vi "Whole Brain Imaging v14.vi"() -> ()   [LabVIEW 2013]
doc: "v4: Added NI DAQ board instead of LabJack\n\nv5: Modified autofocus routine. Changed to triangle wave - AUTOFOCUS DOES NOT WORK ANYMORE\n\nv6: Modified autofocus to work with Triangle Wave. Added Saved Image Number to Lab Jack String."
uses:
  <vilib>/Platform/TimedLoop/XDataNode/timing_clust.ctl
  <vilib>/Platform/TimedLoop/XDataNode/nitl_modes.ctl
  <vilib>/Platform/TimedLoop/XDataNode/wakeup.ctl
  <vilib>/addons/Multicore Analysis and Sparse Matrix/Signal Operation/_sigop/Algorithm Domain.ctl
  <vilib>/event_ctls.llb/eventvkey.ctl
  <vilib>/DAQmx/read.llb/DAQmx Read (Analog 1D DBL NChan 1Samp).vi
  <vilib>/DAQmx/write.llb/DAQmx Write (Analog DBL 1Chan 1Samp).vi
  <vilib>/DAQmx/miscellaneous.llb/DAQmx Fill In Error Info.vi
  <vilib>/addons/Multicore Analysis and Sparse Matrix/Signal Operation/_sigop/1D Convolution (DBL).vi
  <vilib>/addons/Multicore Analysis and Sparse Matrix/Statistics/_statistics/Mean (DBL).vi
  <vilib>/platform/TimedLoop/XDataNode/XDataNode.xnode
  <vilib>/Platform/TimedLoop/XDataNode/XDNodeRunTimeDep.lvlib
  <vilib>/Analysis/NI_AALBase.lvlib
  <vilib>/addons/Multicore Analysis and Sparse Matrix/Signal Operation/NI_MASM_SigOperation.lvlib
  <vilib>/addons/Multicore Analysis and Sparse Matrix/Statistics/NI_MASM_Statistics.lvlib
panel:
  out "Full Cycle 2":dbl[](graph)=[4.263103829970631, 4.263103829970631, 4.263103829970631, 4.263103829970631, 4.263103829970631, 4.263103829970631, 4.263103829970631, 4.263103829970631, 4.263103829970631, 4.263103829970631, 4.263103829970631, 4.263103829970631, 4.263103829970631, 4.263103829970631, 4.263103829970631, 4.263103829970631, 4.263103829970631, 4.263103829970631, 4.263103829970631, 4.263103829970631, 4.263103829970631, 4.263103829970631, 4.263103829970631, 4.263103829970631, 4.263103829970631, 4.263103829970631, 4.263103829970631, 4.263103829970631, 4.263103829970631, 4.263103829970631, 4.263103829970631, 4.263103829970631, 4.263103829970631, 4.263103829970631, 4.263103829970631, 4.263103829970631, 4.263103829970631, 4.263103829970631, 4.263103829970631, 4.263103829970631, 4.263103829970631, 4.263103829970631, 4.263103829970631, 4.263103829970631, 4.263103829970631, 4.263103829970631, 4.263103829970631, 4.263103829970631, 4.263103829970631, 4.263103829970631, 4.263103829970631, 4.263103829970631, 4.263103829970631, 4.263103829970631, 4.263103829970631, 4.263103829970631, 4.263103829970631, 4.263103829970631, 4.263103829970631, 4.263103829970631, 4.263103829970631, 4.263103829970631, 4.263103829970631, 4.263103829970631, 4.263103829970631, 4.263103829970631, 4.263103829970631, 4.263103829970631]
  out "output cluster 2":T1
  out "loopdiff2":i64
  out "output cluster":T2
  in  "Frames 2 wait":i32=1000
  out "Slide":i32(slide) max=1000 scale=-1.0..1000.0
  in  "Latency Check":bool
  out "photodiode":dbl
  in  "Set amplitude":bool
  out "Current Z-ramp Amplitude":dbl=4.0 format="%_3g"
  in  "Focus Knob COM Port":refnum<visa-resource-name>="COM7"
  out "Motorized Focus Knob Found":bool
  out "Turn Up (Counterclockwise)":bool
  out "Turn Down (Clockwise)":bool
  in  "Target Trim (Frames)":dbl
  out "Full Cycle":dbl[](graph)=[4.263103829970631, 4.263103829970631, 4.263103829970631, 4.263103829970631, 4.263103829970631, 4.263103829970631, 4.263103829970631, 4.263103829970631, 4.263103829970631, 4.263103829970631, 4.263103829970631, 4.263103829970631, 4.263103829970631, 4.263103829970631, 4.263103829970631, 4.263103829970631, 4.263103829970631, 4.263103829970631, 4.263103829970631, 4.263103829970631, 4.263103829970631, 4.263103829970631, 4.263103829970631, 4.263103829970631, 4.263103829970631, 4.263103829970631, 4.263103829970631, 4.263103829970631, 4.263103829970631, 4.263103829970631, 4.263103829970631, 4.263103829970631, 4.263103829970631, 4.263103829970631, 4.263103829970631, 4.263103829970631, 4.263103829970631, 4.263103829970631, 4.263103829970631, 4.263103829970631, 4.263103829970631, 4.263103829970631, 4.263103829970631, 4.263103829970631, 4.263103829970631, 4.263103829970631, 4.263103829970631, 4.263103829970631, 4.263103829970631, 4.263103829970631, 4.263103829970631, 4.263103829970631, 4.263103829970631, 4.263103829970631, 4.263103829970631, 4.263103829970631, 4.263103829970631, 4.263103829970631, 4.263103829970631, 4.263103829970631, 4.263103829970631, 4.263103829970631, 4.263103829970631, 4.263103829970631, 4.263103829970631, 4.263103829970631, 4.263103829970631, 4.263103829970631]
  out "Peak Position":dbl=nan
  out "Target":dbl=17.0
  in  "AutoFocus":u16(ring)=1 items=["Both", "Red", "Green"]
  out "Stage Y":i32=-50106
  out "Stage X":i32=-79365
  out "TotalFramesHidden":i32=32650
  out "Half Cycle":dbl[](graph)
  out "Saved Images Hidden":i32=28989
  in  "Z Ramp\nFrequency (Hz)\n[Must Quit To Update]":dbl=3.0
  in  "Latency Shift (Frames)":i16 max=5000 step=1
  out "sCMOS Image":u16[][](graph)
  in  "ROI":T3={"Horizontal Offset"=418, "Vertical Offset"=818, "Horizontal Width"=1200, "Vertical Width"=600}
  in  "Exposure (ms)":dbl=5.0
  in  "Binning":u16(ring)=1 items=["1x1"=1, "2x2"=2, "4x4"=4]
  out "Read Frames":i32=32581
  in  "Save Image":bool
  out "Written":string="\r\r---------------------  NEW FILE  ---------------------\rO:\\20150616\\BrainScanner20150616_111602\r\r6/16/2015 11:17 AM\rignore first 17000 frames\n\r\r6/16/2015 11:17 AM\runtil third flash\n\r\r6/16/2015 11:18 AM\rbecause my autofocus gain was off\n\r\r6/16/2015 11:18 AM\rworm isn't very active\n\r\r"
  in  "Comments":string
  out "User Comments  File":path=path "O:/20150616/Comments.txt"
  in  "Zero DC Offset":bool
  out "Quit Pushed?":bool=TRUE
  in  "Autofocus Gain":dbl=0.03
  out "Camera Trigger":dbl=0.00885779825410911 format="%.6f"
  out "Camera Frame File":path=path "O:/20150616/BrainScanner20150616_111602/CameraFrameData.txt"
  out "FxnGen Sync":dbl=0.14061238584404193 format="%.6f"
  out "Z Sensor":dbl=6.145352387169191 format="%.6f"
  out "LabJack File":path=path "O:/20150616/BrainScanner20150616_111602/LabJackData.txt"
  out "Dropped Frames":i32=68
  out "Current Image":u16[][](array[numeric])
  out "Image StDev":dbl=4.263103829970631
  out "FuncGen Voltage":dbl=5.836089361558744 format="%.6f"
  out "Z-ramp DC Offset":dbl=nan
  in  "Autofocus":bool
  out "sCMOS Camera Image File":path=path "O:/20150616/BrainScanner20150616_111602/sCMOS_Frames_U16_1024x1024.dat"
  in  "Z-ramp":bool
  in  "Z-ramp Amplitude (4) (Votls)":dbl=4.0 format="%_3g"
  out "Elapsed Time":string="0 : 2 : 43.5"
  out "Saved Frames":i32=28988
  out "Save Directory":path=path "O:/20150616/BrainScanner20150616_111602"
  out "Camera Info":string="C11440-22C; S/N: 751007; 2.50.A"
  out "Total Frames":i32=32649
  in  "Quit":bool
  # "Note: For unknwon reasons, the latency varies from session-to-session and also varies with sweep frequency.\nTo measure and compensate for the latency:\n1) Set Gain to 0 and turn on autofocus.\n2) While recording from bead slide,  adjust  focus knob so that only one peak appears in Full Cycle graph. Beads should be at extreme edge of scan range.\n3)Adjust the latency shift until the single peak appears split on both sides of the graph. \n4) Adjust the focus knob so the beads are back in the center of the scan range\n5) Make the autofocus gain non-zero (e.g. 0.1). You will likely need to try both positive and negative values."
  # "ChangeLog:\nv14. Andy tries to add in the  focus knob controller"
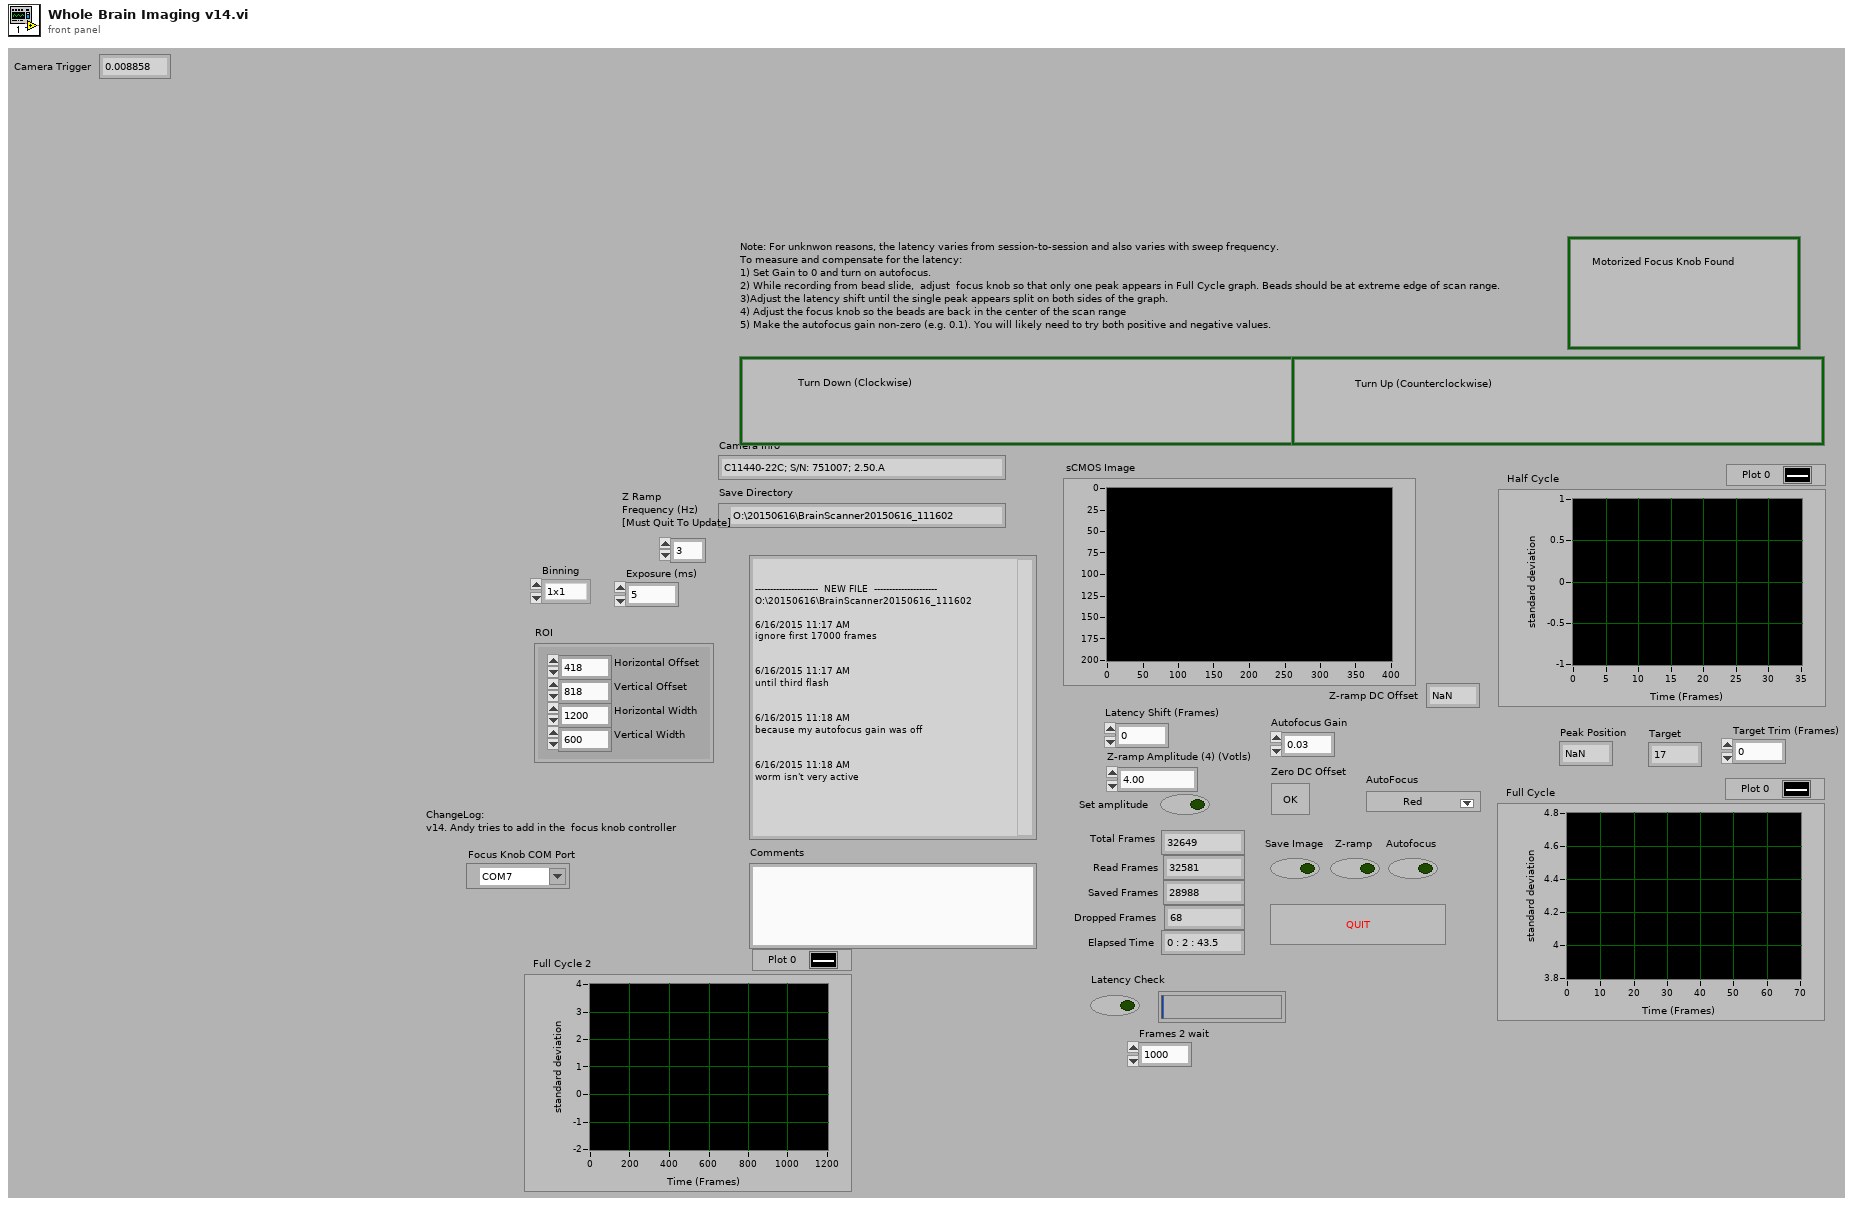
[diagram p1: front panel]
types:
  T1 = cluster{"Waveform":dbl, "standard deviation":dbl}
  T2 = cluster{"Actual Start [i]":i64, "standard deviation":dbl}
  T3 = cluster{"Horizontal Offset":i32, "Vertical Offset":i32, "Horizontal Width":i32, "Vertical Width":i32}
  T4 = enum8{"Enabled", "Disabled", "Disabled and Grayed Out"}
  T5 = typedef "XDNodeRunTimeDep.lvlib/timing_clust.ctl" = cluster{"Expected End [f-1]":u64, "Actual End [f-1]":u64, "Finished Late? [f-1]":bool, "Expected End [i-1]":u64, "Actual End [i-1]":u64, "Finished Late? [i-1]":bool, "Expected Start [i]":u64, "Actual Start [i]":u64, "Expected Start [f]":u64, "Actual Start [f]":u64, "Source Name":string, "Structure Name":string, "Period":i64, "Deadline":i64, "Offset":i64, "Start":i64, "Priority":i32, "Timeout":i32, "Mode":T6, "Wakeup Reason":T7, "Error":errorcluster, "Source Type":string, "Secondary Source Type":string, "Global End Time":u64, "Global Start Time":u64, "Frame Duration":u64, "Iteration Duration":u64, "Assigned CPU":i32, "I/O Scan Engine Mode":u32}
  T6 = typedef "XDNodeRunTimeDep.lvlib/nitl_modes.ctl" = enum32{"No Change", "Process missed periods, maintain original phase", "Discard missed periods, maintain original phase", "Process missed periods, ignore original phase", "Discard missed periods, ignore original phase"}
  T7 = typedef "XDNodeRunTimeDep.lvlib/wakeup.ctl" = enum32{"Normal", "Aborted", "Asynchronous wakeup", "Timing source error", "Timed loop error", "Timeout"}
  T8 = typedef "NI_MASM_SigOperation.lvlib/Algorithm Domain.ctl" = i32
  T9 = enum16{"open", "replace", "create", "open or create", "replace or create", "replace or create with confirmation"}
  T10 = cluster{"height":u32, "width":u32, "datatype":u32}
  T11 = cluster{"Mode":u32, "Polarity":u32, "Period":dbl, "Delay":dbl}
  T12 = typedef "eventvkey.ctl" = enum16{"ASCII", "Enter", "Return", "Shift", "Ctrl", "Alt", "Cmd", "Opt", "Caps", "NumLock", "Clear", "Break", "Up", "Down", "Left", "Right", "Insert", "Delete", "Home", "End", "PageUp", "PageDown", "Escape", "Help", "Pause", "ScrollLock", "F1", "F2", "F3", "F4", "F5", "F6", "F7", "F8", "F9", "F10", "F11", "F12", "F13", "F14", "F15", "F16", "F17", "F18", "F19", "F20", "F21", "F22", "F23", "F24", "Play", "VolumeUp", "VolumeDown", "Mute", "Two Byte Char"}
  T13 = enum16{"big-endian, network order", "native, host order", "little-endian"}
  T14 = cluster{"standard deviation":dbl, "Waveform":dbl}
  T15 = cluster{"millisecond timer value":u32, "standard deviation":dbl}
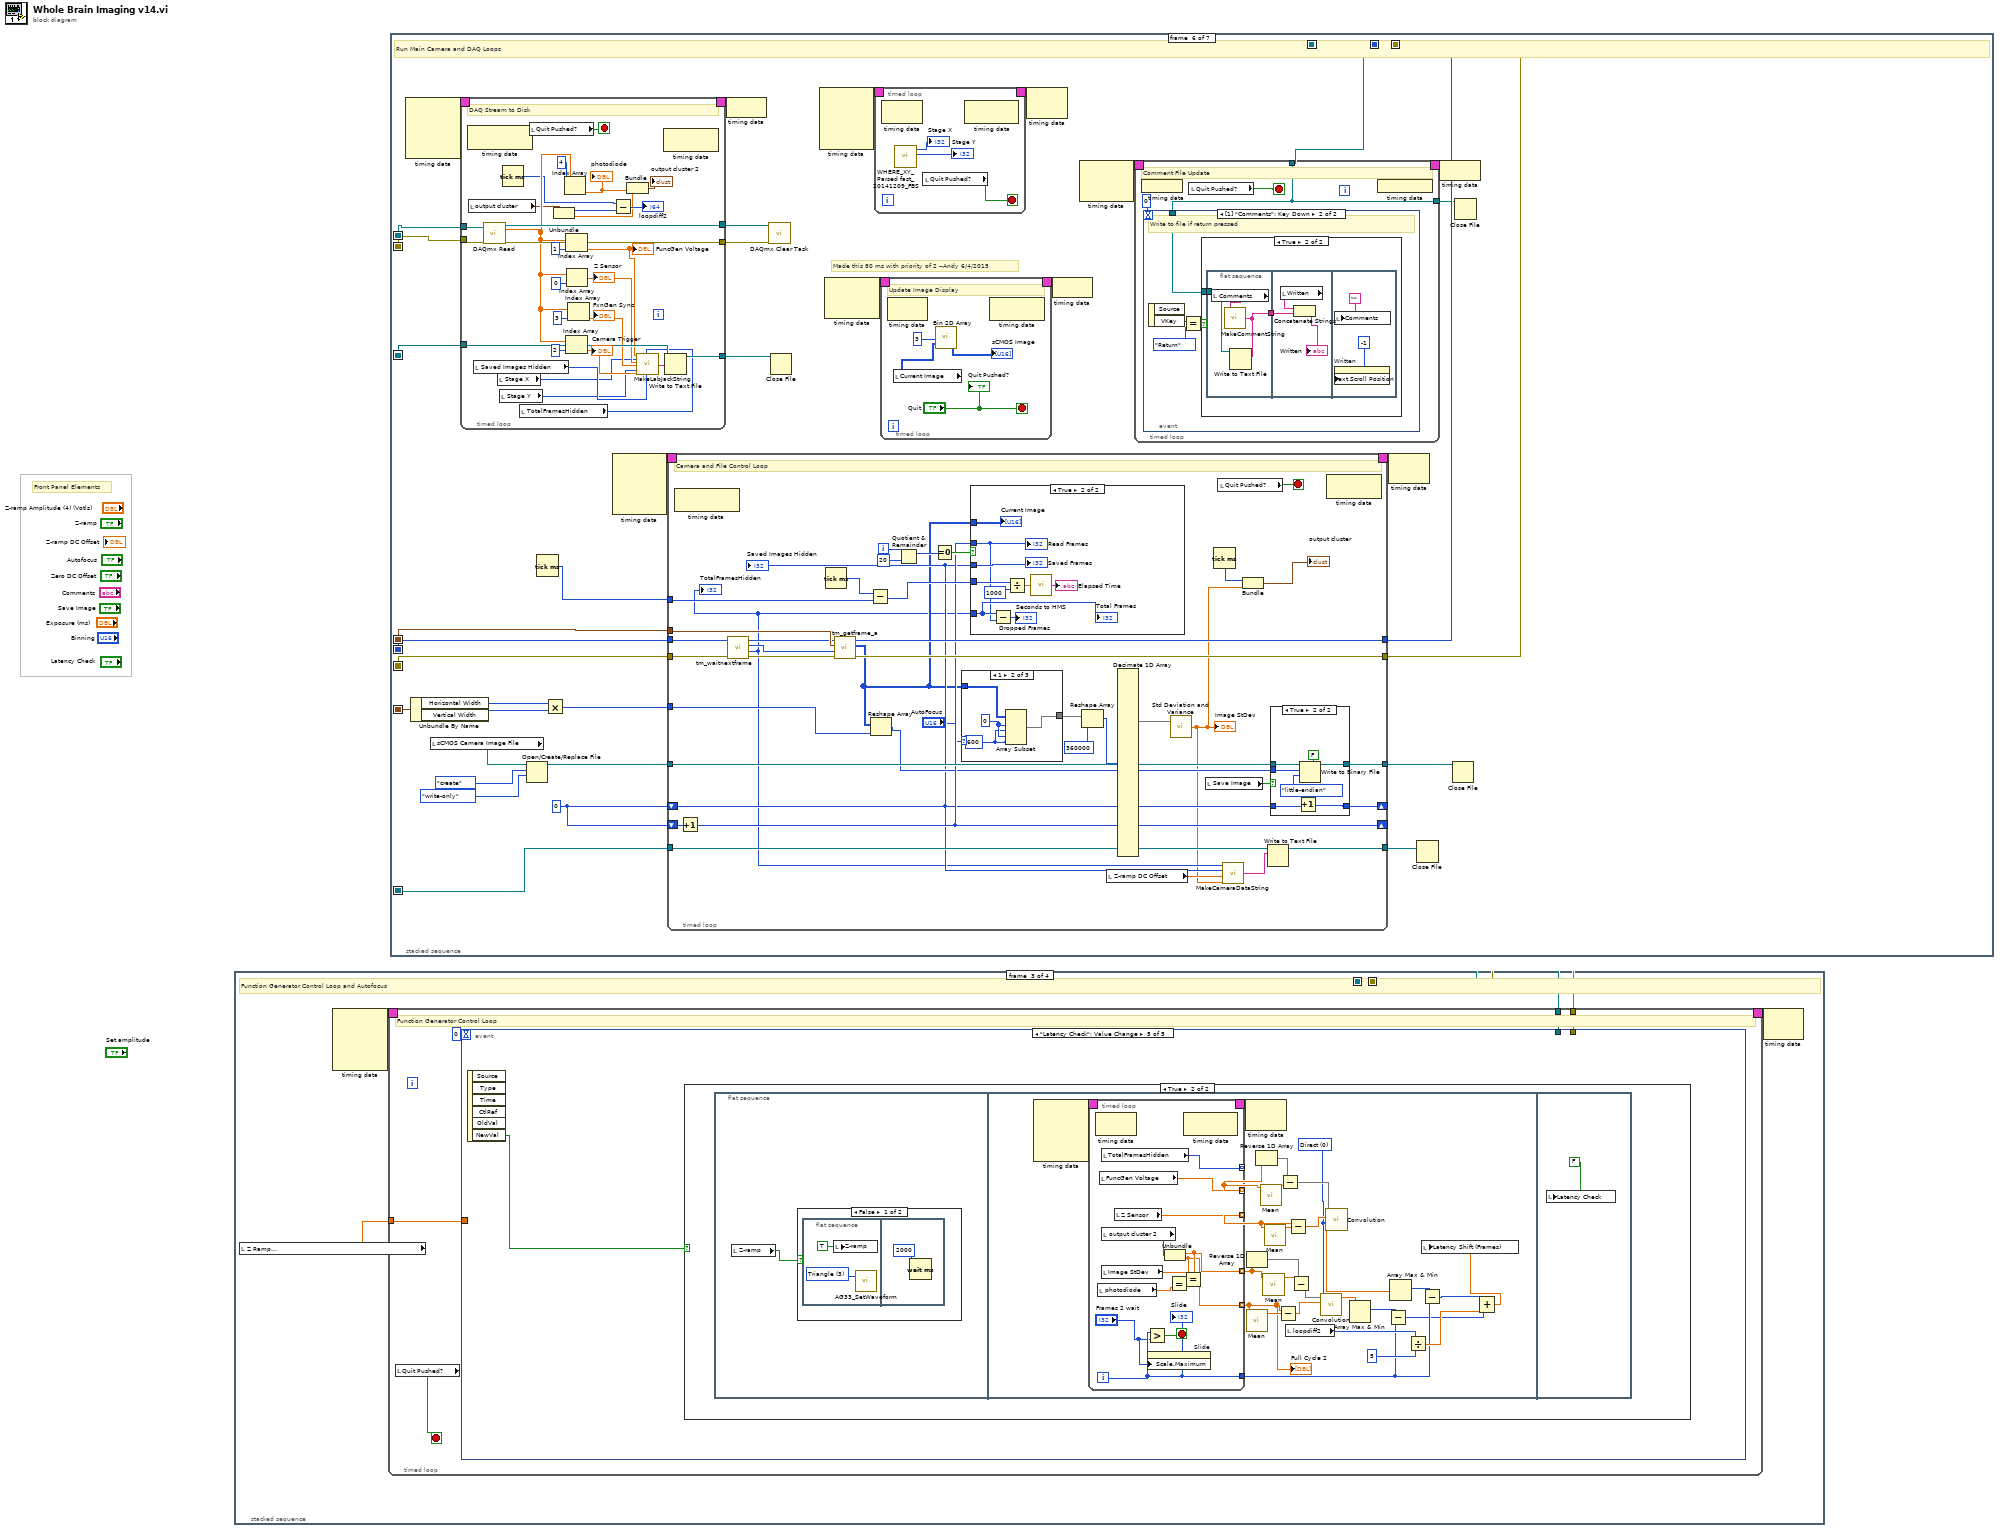
[diagram p0: block diagram]
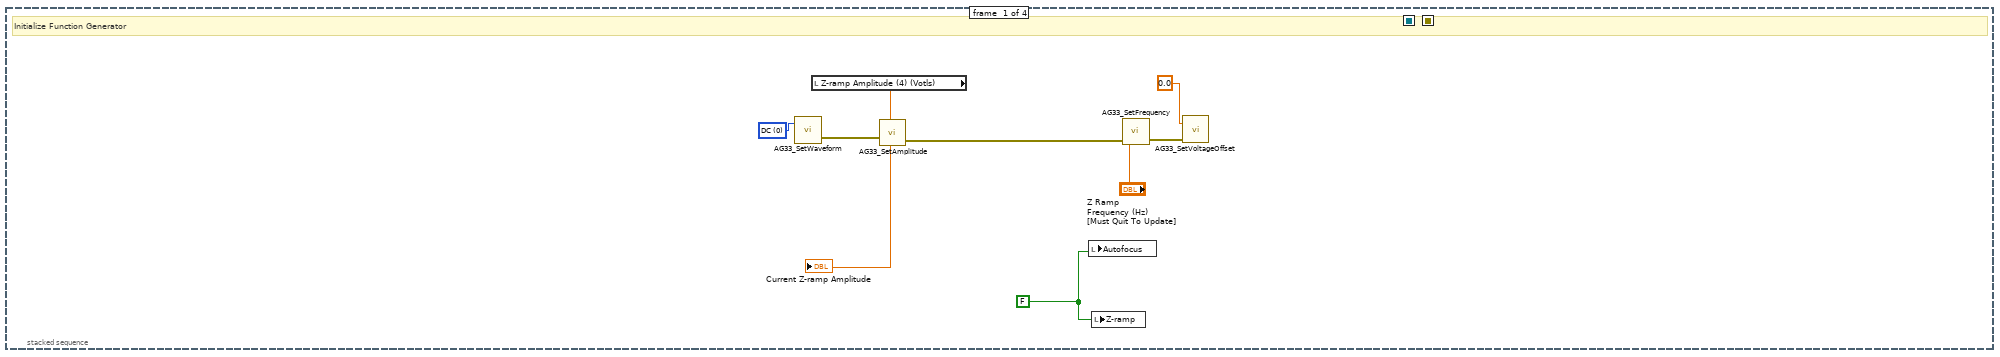
[diagram p2: hidden frame]
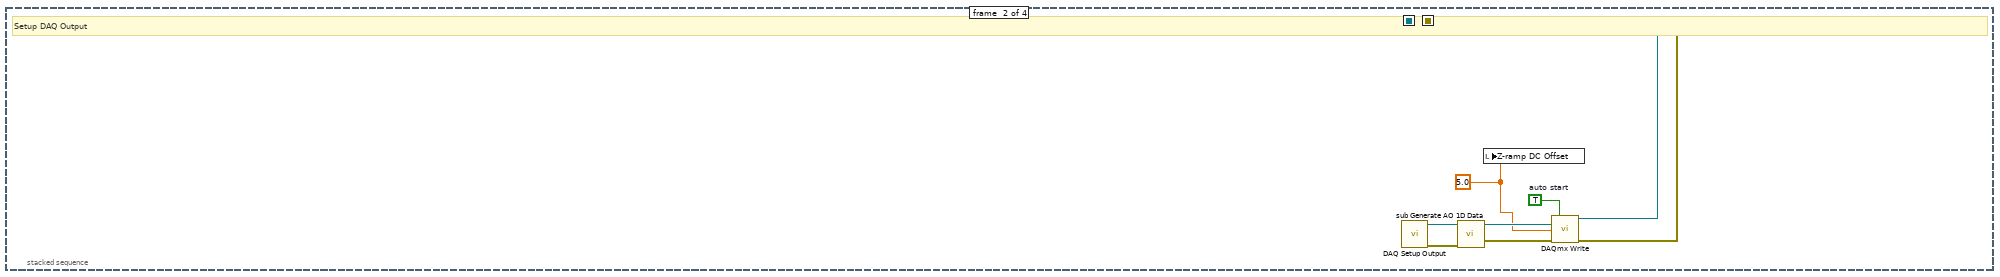
[diagram p3: hidden frame]
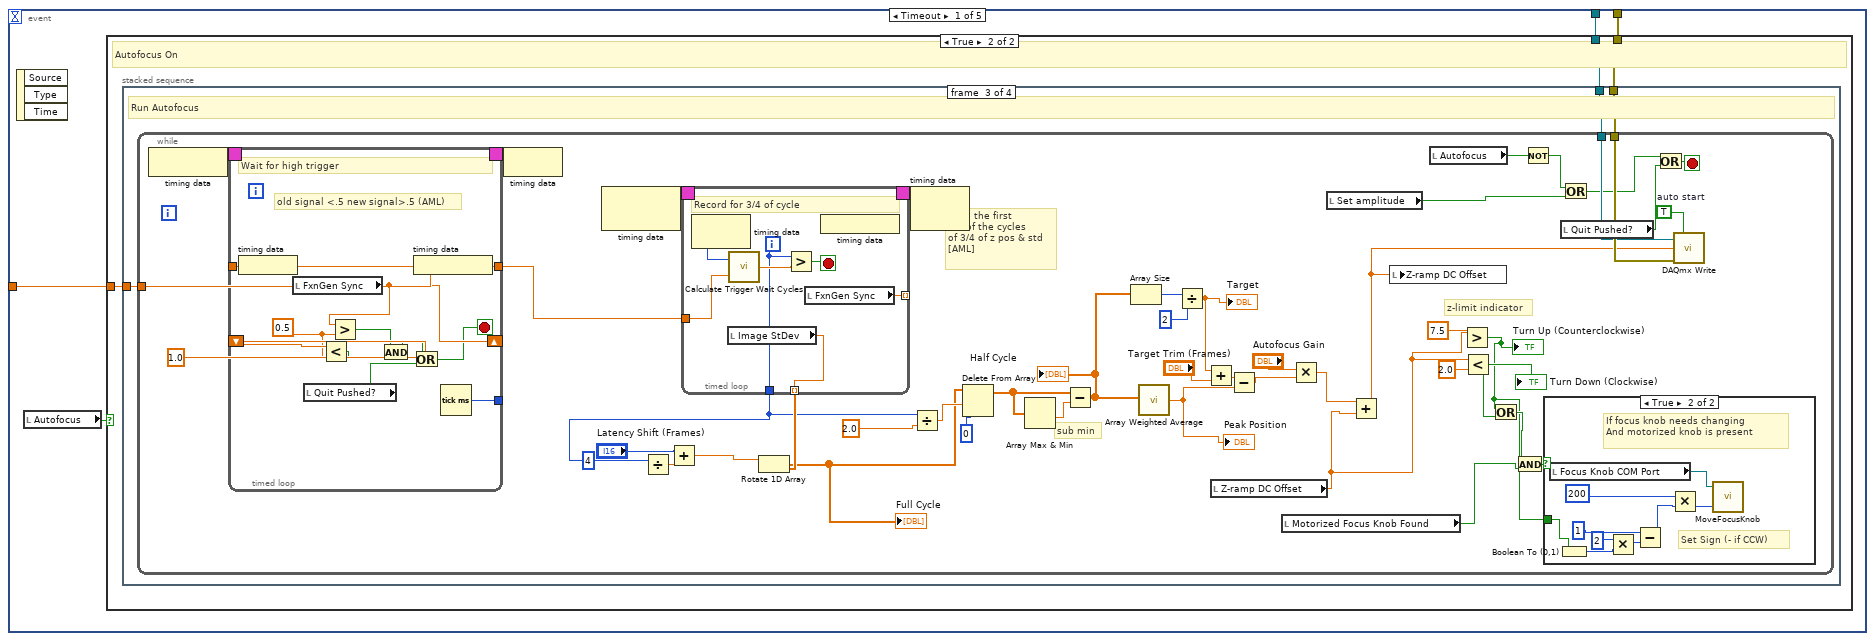
[diagram p4: hidden frame]
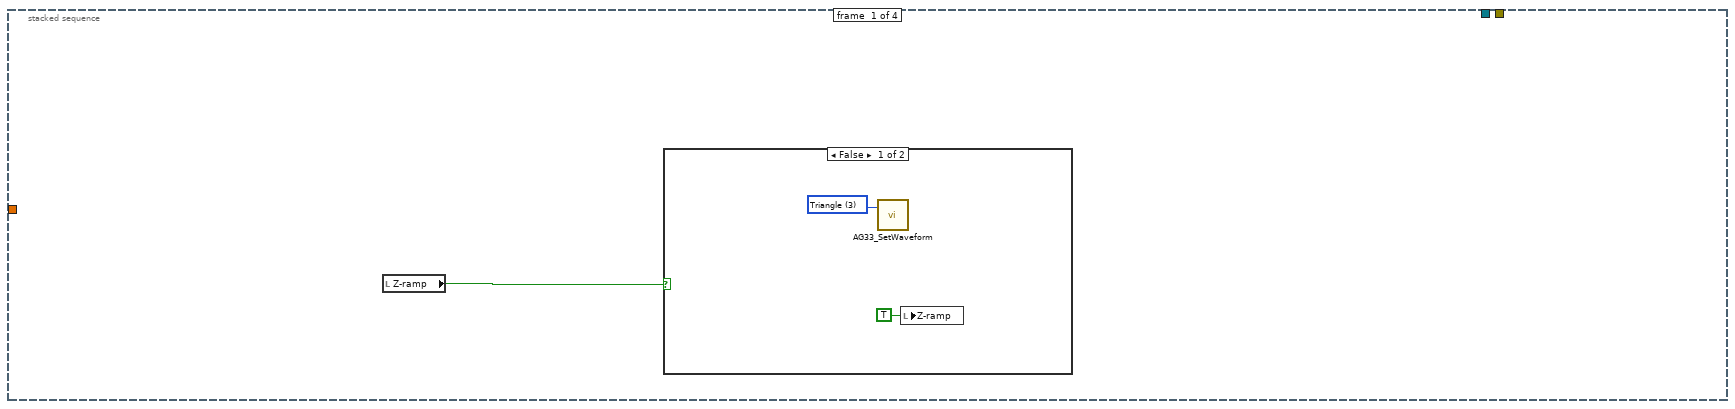
[diagram p6: hidden frame]
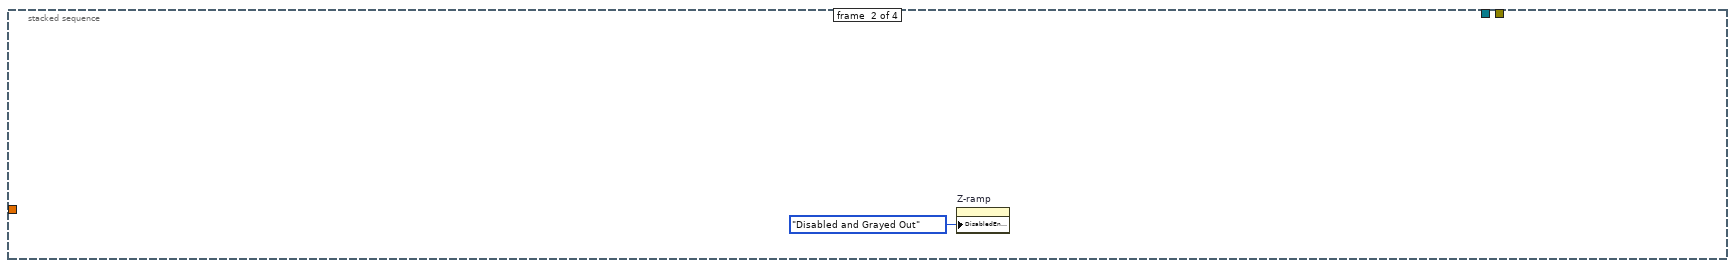
[diagram p8: hidden frame]
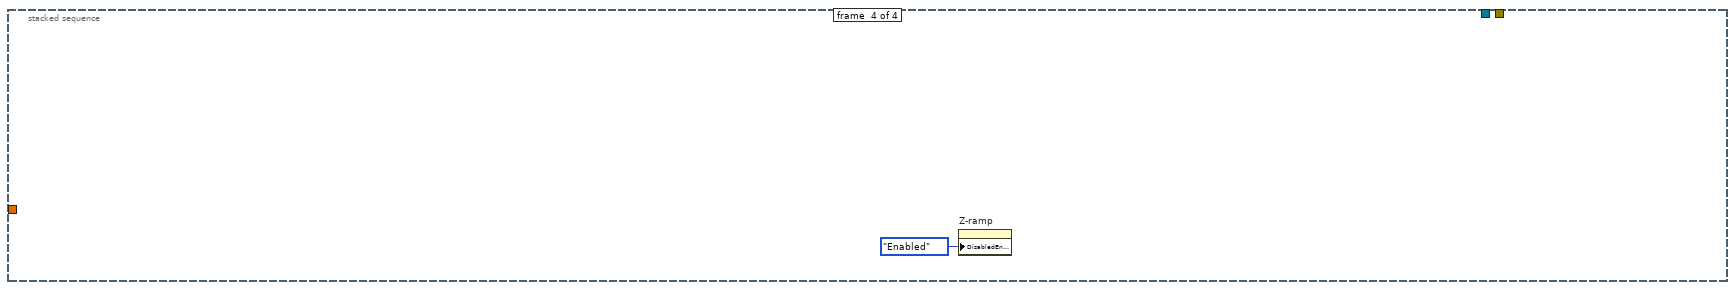
[diagram p10: hidden frame]
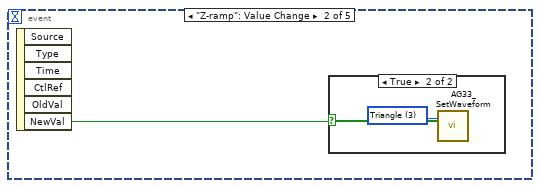
[diagram p11: hidden frame]
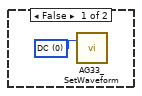
[diagram p12: hidden frame]
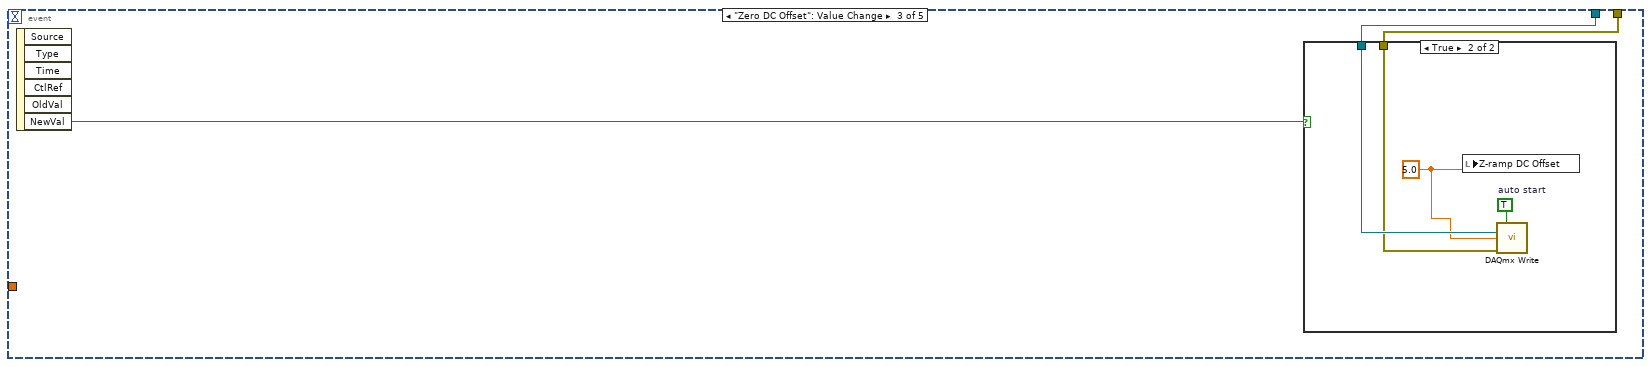
[diagram p13: hidden frame]
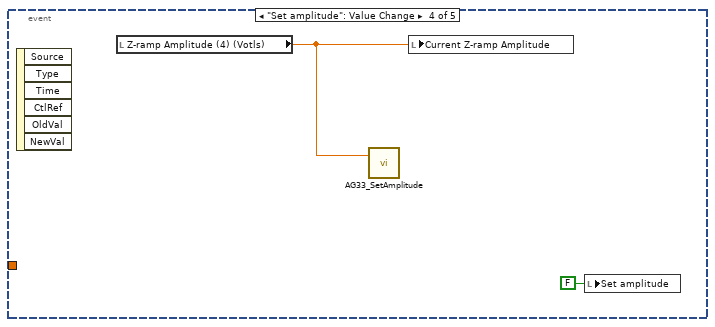
[diagram p15: hidden frame]
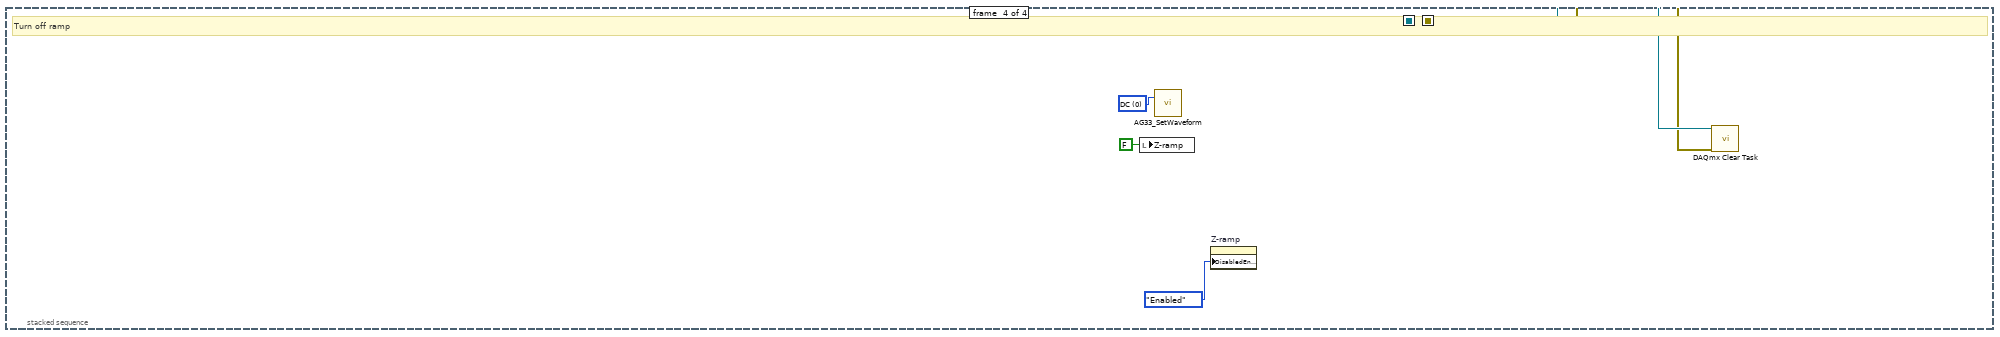
[diagram p18: hidden frame]
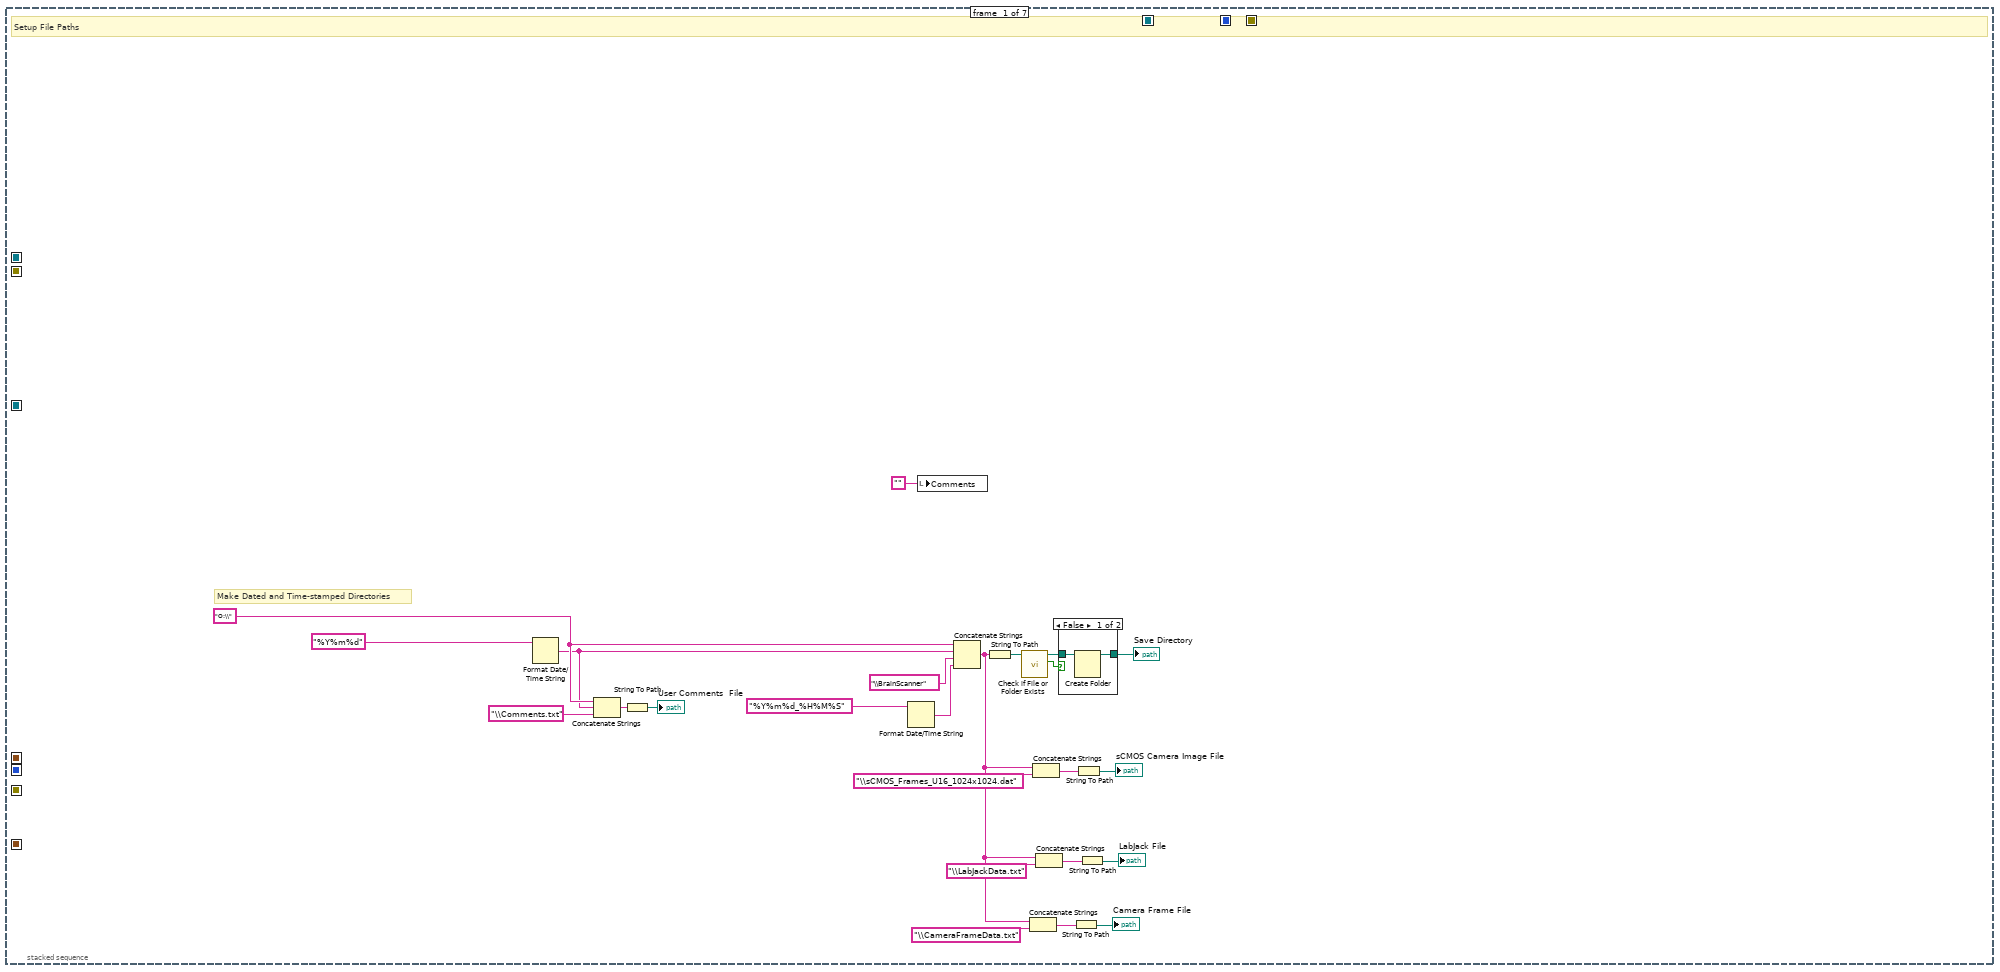
[diagram p19: hidden frame]
diagram:
  # "Front Panel Elements"
  n1 = stacked-sequence {
    seq-local: [_ w10 _ _] -> [_ _ w19 w191]
    seq-local: [_ w11 _ _] -> [_ _ w18 w190]
    frame #0 {
      w2 = FALSE ("stop")
      w8 = u16 0 items=["DC", "Sine", "Square", "Triangle", "Ramp", "Pulse", "Noise", "Sinc", "Negative Ramp", "Exponential Rise", "Exponential Fall", "Cardiac"] ("Waveform Function (1: Sine)")
      # "Initialize Function Generator"
      n2 = call "AG33_SetWaveform.vi"("Waveform Function (1: Sine)"=w8) -> ("error out"=w6:errorcluster)  [unwired: 2 in]
      n3 = local read "Z-ramp Amplitude (4) (Votls)"() -> (w7:dbl)
      "Current Z-ramp Amplitude" <- w7
      n4 = call "AG33_SetAmplitude.vi"("error in (no error)"=w6, "Amplitude (Vpp)"=w7) -> ("error out"=w5:errorcluster)  [unwired: 1 in]
      n5 = local write "Autofocus"(w2) -> ()
      n6 = local write "Z-ramp"(w2) -> ()
      n7 = call "AG33_SetFrequency.vi"("error in (no error)"=w5, "Frequency (Hz)"="Z Ramp\nFrequency (Hz)\n[Must Quit To Update]") -> ("error out"=w4:errorcluster)  [unwired: 1 in]
      n8 = call "AG33_SetVoltageOffset.vi"("error in (no error)"=w4, "DC Offset (0.00 V)"=0.0) -> ()  [unwired: 1 in, 1 out]
    }
    frame #1 {
      w9 = 5.0 ("DC Offset (0.00 V)")
      w14 = TRUE  # auto start
      # "Setup DAQ Output"
      n9 = call "DAQ Setup Output.vi"() -> ("error out"=w16:errorcluster, "task out"=w15:refnum<k21>)  [unwired: 10 in]
      n10 = call <vilib>:"sub Generate AO 1D Data.vi"("error in"=w16, "task in"=w15) -> ("error out"=w13:errorcluster, "task out"=w12:refnum<k21>)  [unwired: 7 in, 1 out]
      n11 = local write "Z-ramp DC Offset"(w9) -> ()
      n12 = call-poly <vilib>:"DAQmx Write.vi"("task/channels in"=w12, "auto start"=w14, "data"=w9, "error in"=w13) -> ("task out"=w10:refnum<k21>, "error out"=w11:errorcluster)  [unwired: 9 in, 1 out]
    }
    frame #2 {
      # "Function Generator Control Loop and Autofocus"
      n13 = local read "Z Ramp\nFrequency (Hz)\n[Must Quit To Update]"() -> (w17:dbl)
      n14 = node-c288() -> (w21:T5)  [unwired: 4 in]
      n15 = timed-loop {
        timing: w21 -> [_]
        timing-out: [_] -> w20
        tunnel: w19 -> [w24]
        tunnel: w18 -> [w23]
        tunnel: w17 -> [w22]
        stop <- w25 stop-if-true
        # "Function Generator Control Loop"
        n16 = local read "Quit Pushed?"() -> (w25:bool)
        n17 = event shown="[4] \"Latency Check\": Value Change" {
          selector: _ -> [_ _ _ _ _]
          dyn-events: _ -> [_ _ _ _ _]
          timeout: 0 -> [_ _ _ _ _]
          tunnel: w24 -> [w29 _ w128 _ _]
          tunnel: w23 -> [w28 _ w127 _ _]
          tunnel: w22 -> [w27 _ _ _ _]
          event Timeout {
            n18 = event-data() -> ()  [unwired: 1 in, 3 out]
            n19 = local read "Autofocus"() -> (w30:bool)
            n20 = case shown="True" w30 {
              tunnel: w29 -> [_ w33]
              tunnel: w28 -> [_ w32]
              tunnel: w27 -> [_ w31]
              frame False {
                # "Autofocus Off"
              }
              frame True {
                # "Autofocus On"
                n21 = stacked-sequence {
                  tunnel: w33 -> [_ _ w40 _]
                  tunnel: w32 -> [_ _ w39 _]
                  tunnel: w31 -> [_ _ w38 _]
                  frame #0 {
                    n22 = local read "Z-ramp"() -> (w34:bool)
                    n23 = case shown="False" w34 {
                      frame False {
                        w36 = u16 3 items=["DC", "Sine", "Square", "Triangle", "Ramp", "Pulse", "Noise", "Sinc", "Negative Ramp", "Exponential Rise", "Exponential Fall", "Cardiac"] ("Waveform Function (1: Sine)")
                        n24 = call "AG33_SetWaveform.vi"("Waveform Function (1: Sine)"=w36) -> ()  [unwired: 2 in, 1 out]
                        n25 = local write "Z-ramp"(TRUE ("Z-ramp")) -> ()
                      }
                      frame True {
                      }
                    }
                  }
                  frame #1 {
                    n26 = property on="Z-ramp" class="Bool (strict)"("DisabledEnum"=T4."Disabled and Grayed Out" ("Disabled")) -> ()  [unwired: 2 in, 2 out]
                  }
                  frame #2 {
                    # "Run Autofocus"
                    n27 = while {
                      tunnel: w40 -> [w85]
                      tunnel: w39 -> [w87]
                      tunnel: w38 -> [w84]
                      stop <- w86 stop-if-true
                      w77 = TRUE  # auto start
                      # "z-limit indicator"
                      # "sub min"
                      # "Take the first\n3/4 of the cycles\nof 3/4 of z pos & std\n[AML]"
                      n28 = node-c288() -> (w81:T5)
                      n29 = timed-loop {
                        timing: w81 -> [_]
                        timing-out: [_] -> w80
                        shift-right: [w101] -> _
                        shift-left: 1.0 -> [w104]
                        tunnel: w84 -> [w106]
                        tunnel: [w106] -> w46
                        tunnel: [w97] -> _
                        stop <- w98 stop-if-true
                        w102 = 0.5
                        # "old signal <.5 new signal>.5 (AML)"
                        # "Wait for high trigger"
                        n30 = node-c288() -> ()  [unwired: 1 in]
                        n31 = local read "FxnGen Sync"() -> (w101:dbl)
                        n32 = local read "Quit Pushed?"() -> (w99:bool)
                        n33 = Less?(x=w104, y=w102) -> (x < y?=w105:bool)
                        n34 = Greater?(x=w101, y=w102) -> (0:w103:bool)
                        n35 = And(x=w103, y=w105) -> (x .and. y?=w100:bool)
                        n36 = Or(x=w100, y=w99) -> (x .or. y?=w98:bool)
                        n37 = node-c288() -> ()  [unwired: 1 out]
                        n38 = Tick Count (ms)() -> (millisecond timer value=w97:u32)
                      }
                      n39 = node-c288(w80) -> ()
                      n40 = node-c288() -> (w83:T5)  [unwired: 1 in]
                      n41 = timed-loop {
                        tunnel: [w117] -> w65 mode=indexing
                        timing: w83 -> [_]
                        timing-out: [_] -> w82
                        tunnel: w46 -> [w115]
                        tunnel: [w113] -> w43
                        tunnel: [w111] -> _ mode=indexing
                        i -> [w113]
                        stop <- w112 stop-if-true
                        # "Record for 3/4 of cycle"
                        n42 = node-c288() -> (w116:i64)  [unwired: 1 in]
                        n43 = local read "Image StDev"() -> (w117:dbl)
                        n44 = call "Calculate Trigger Wait Cycles.vi"("Frequency (Hz)"=w115, "Period (ms)"=w116) -> ("Cycles to Wait"=w114:dbl)
                        n45 = Greater?(x=w113, y=w114) -> (0:w112:bool)
                        n46 = local read "FxnGen Sync"() -> (w111:dbl)
                        n47 = node-c288() -> ()  [unwired: 1 out]
                      }
                      n48 = Divide(x=w43, y=4) -> (x/y=w44:dbl)
                      n49 = Add(x="Latency Shift (Frames)", y=w44) -> (x+y=w41:dbl)
                      n50 = Rotate 1D Array(1:w65, 2:w41) -> (0:w64:dbl[])
                      "Full Cycle" <- w64
                      n51 = node-c288(w82) -> ()  [unwired: 1 out]
                      n52 = Divide(x=w43, y=2.0) -> (x/y=w67:dbl)
                      n53 = Delete From Array(array=w64, length=w67, index=0 ("length")) -> (array with subset deleted=w76:dbl[])  [unwired: 1 out]
                      n54 = Array Max & Min(array=w76) -> (min value=w75:dbl)  [unwired: 3 out]
                      n55 = Subtract(x=w76, y=w75) -> (x-y=w59:dbl[])
                      "Half Cycle" <- w59
                      n56 = Array Size(array=w59) -> (size(s)=w72:i32)
                      n57 = call "Array Weighted Average.vi"("Input Array"=w59) -> ("Weighted Average Index"=w58:dbl)
                      "Peak Position" <- w58
                      n58 = Divide(x=w72, y=2) -> (x/y=w60:dbl)
                      "Target" <- w60
                      n59 = Add(x=w60, y="Target Trim (Frames)") -> (x+y=w62:dbl)
                      n60 = local read "Z-ramp DC Offset"() -> (w55:dbl)
                      n61 = Subtract(x=w62, y=w58) -> (x-y=w63:dbl)
                      n62 = local read "Motorized Focus Knob Found"() -> (w51:bool)
                      n63 = Multiply(x="Autofocus Gain", y=w63) -> (x*y=w69:dbl)
                      n64 = local read "Set amplitude"() -> (w47:bool)
                      n65 = Add(x=w69, y=w55) -> (x+y=w68:dbl)
                      n66 = local write "Z-ramp DC Offset"(w68) -> ()
                      n67 = local read "Autofocus"() -> (w79:bool)
                      n68 = Greater?(x=w55, y=7.5) -> (0:w50:bool)
                      "Turn Up (Counterclockwise)" <- w50
                      n69 = Less?(x=w55, y=2.0) -> (x < y?=w54:bool)
                      "Turn Down (Clockwise)" <- w54
                      n70 = Or(x=w50, y=w54) -> (x .or. y?=w52:bool)
                      n71 = And(x=w52, y=w51) -> (x .and. y?=w53:bool)
                      n72 = Not(x=w79) -> (.not. x?=w49:bool)
                      n73 = case shown="True" w53 {
                        tunnel: w50 -> [_ w93]
                        frame False {
                        }
                        frame True {
                          # "Set Sign (- if CCW)"
                          # "If focus knob needs changing\nAnd motorized knob is present"
                          n74 = local read "Focus Knob COM Port"() -> (w96:refnum<visa-resource-name>)
                          n75 = Boolean To (0,1)(Boolean=w93) -> (0, 1=w89:i16)
                          n76 = Multiply(x=2, y=w89) -> (x*y=w91:i32)
                          n77 = Subtract(x=1, y=w91) -> (x-y=w88:i32)
                          n78 = Multiply(x=200 ("Hunderdths of of Microns"), y=w88) -> (x*y=w95:i32)
                          n79 = call "MoveFocusKnob.vi"("VISA resource name"=w96, "Hunderdths of of Microns"=w95) -> ()  [unwired: 2 in, 3 out]
                        }
                      }
                      n80 = Or(x=w49, y=w47) -> (x .or. y?=w48:bool)
                      n81 = local read "Quit Pushed?"() -> (w78:bool)
                      n82 = Or(x=w48, y=w78) -> (x .or. y?=w86:bool)
                      n83 = call-poly <vilib>:"DAQmx Write.vi"("task/channels in"=w85, "auto start"=w77, "data"=w68, "error in"=w87) -> ()  [unwired: 9 in, 3 out]
                    }
                  }
                  frame #3 {
                    n84 = property on="Z-ramp" class="Bool (strict)"("DisabledEnum"=T4."Enabled" ("Disabled")) -> ()  [unwired: 2 in, 2 out]
                  }
                }
              }
            }
          }
          event "Z-ramp": Value Change {
            n85 = event-data() -> ("NewVal"=w124:bool)  [unwired: 1 in, 5 out]
            n86 = case shown="True" w124 {
              frame False {
                w125 = u16 0 items=["DC", "Sine", "Square", "Triangle", "Ramp", "Pulse", "Noise", "Sinc", "Negative Ramp", "Exponential Rise", "Exponential Fall", "Cardiac"] ("Waveform Function (1: Sine)")
                n87 = call "AG33_SetWaveform.vi"("Waveform Function (1: Sine)"=w125) -> ()  [unwired: 2 in, 1 out]
              }
              frame True {
                w126 = u16 3 items=["DC", "Sine", "Square", "Triangle", "Ramp", "Pulse", "Noise", "Sinc", "Negative Ramp", "Exponential Rise", "Exponential Fall", "Cardiac"] ("Waveform Function (1: Sine)")
                n88 = call "AG33_SetWaveform.vi"("Waveform Function (1: Sine)"=w126) -> ()  [unwired: 2 in, 1 out]
              }
            }
          }
          event "Zero DC Offset": Value Change {
            n89 = event-data() -> ("NewVal"=w129:bool)  [unwired: 1 in, 5 out]
            n90 = case shown="True" w129 {
              tunnel: w128 -> [_ w132]
              tunnel: w127 -> [_ w131]
              frame False {
              }
              frame True {
                w133 = TRUE  # auto start
                w130 = 5.0 ("DC Offset (0.00 V)")
                n91 = local write "Z-ramp DC Offset"(w130) -> ()
                n92 = call-poly <vilib>:"DAQmx Write.vi"("task/channels in"=w132, "auto start"=w133, "data"=w130, "error in"=w131) -> ()  [unwired: 9 in, 3 out]
              }
            }
          }
          event "Set amplitude": Value Change {
            n93 = event-data() -> ()  [unwired: 1 in, 6 out]
            n94 = local read "Z-ramp Amplitude (4) (Votls)"() -> (w135:dbl)
            n95 = call "AG33_SetAmplitude.vi"("Amplitude (Vpp)"=w135) -> ()  [unwired: 2 in, 1 out]
            n96 = local write "Current Z-ramp Amplitude"(w135) -> ()
            n97 = local write "Set amplitude"(FALSE ("Set amplitude")) -> ()
          }
          event "Latency Check": Value Change {
            n98 = event-data() -> ("NewVal"=w136:bool)  [unwired: 1 in, 5 out]
            n99 = case shown="True" w136 {
              frame False {
              }
              frame True {
                n100 = flat-sequence {
                  frame #0 {
                    n101 = local read "Z-ramp"() -> (w137:bool)
                    n102 = case shown="False" w137 {
                      frame False {
                        n103 = flat-sequence {
                          frame #0 {
                            w139 = u16 3 items=["DC", "Sine", "Square", "Triangle", "Ramp", "Pulse", "Noise", "Sinc", "Negative Ramp", "Exponential Rise", "Exponential Fall", "Cardiac"] ("Waveform Function (1: Sine)")
                            n104 = local write "Z-ramp"(TRUE ("Z-ramp")) -> ()
                            n105 = call "AG33_SetWaveform.vi"("Waveform Function (1: Sine)"=w139) -> ()  [unwired: 2 in, 1 out]
                          }
                          frame #1 {
                            n106 = Wait (ms)(milliseconds to wait=u32 2000) -> ()  [unwired: 1 out]
                          }
                        }
                      }
                      frame True {
                      }
                    }
                  }
                  frame #1 {
                    w147 = T8 0 items=["Direct", "Frequency Domain"] ("algorithm")
                    n107 = node-c288() -> (w168:T5)  [unwired: 4 in]
                    n108 = timed-loop {
                      timing: w168 -> [_]
                      timing-out: [_] -> w167
                      tunnel: [w177] -> w160 mode=indexing
                      tunnel: [w176] -> w163 mode=indexing
                      tunnel: [w178] -> _ mode=indexing
                      tunnel: [w175] -> w144
                      tunnel: [w172] -> w142 mode=indexing
                      tunnel: [w170] -> w141 mode=indexing
                      i -> [w175]
                      stop <- w179 stop-if-true
                      n109 = node-c288() -> ()  [unwired: 1 in, 1 out]
                      n110 = local read "photodiode"() -> (w169:dbl)
                      n111 = local read "FuncGen Voltage"() -> (w177:dbl)
                      n112 = local read "TotalFramesHidden"() -> (w178:i32)
                      n113 = local read "Image StDev"() -> (w171:dbl)
                      n114 = local read "output cluster 2"() -> (w173:T1)
                      n115 = local read "Z Sensor"() -> (w176:dbl)
                      n116 = Greater?(x=w175, y="Frames 2 wait") -> (0:w179:bool)
                      n117 = property on="Slide" class="Slide (strict)"("Scale.Maximum"="Frames 2 wait") -> ()  [unwired: 2 in, 2 out]
                      n118 = Unbundle(w173) -> ("Waveform"=w172:dbl, "standard deviation"=w170:dbl)
                      n119 = Equal?(x=w170, y=w169) -> ()  [unwired: 1 out]
                      n120 = Equal?(x=w172, y=w171) -> ()  [unwired: 1 out]
                      n121 = node-c288() -> ()  [unwired: 1 in, 1 out]
                      "Slide" <- w175
                    }
                    "Full Cycle 2" <- w141
                    n122 = node-c288(w167) -> ()  [unwired: 1 out]
                    n123 = Reverse 1D Array(array=w142) -> (reversed array=w152:dbl[])
                    n124 = call-poly <vilib>:"Mean.vi"("X"=w141) -> ("mean"=w149:dbl)  [unwired: 9 in, 1 out]
                    n125 = Reverse 1D Array(array=w160) -> (reversed array=w159:dbl[])
                    n126 = call-poly <vilib>:"Mean.vi"("X"=w160) -> ("mean"=w165:dbl)  [unwired: 9 in, 1 out]
                    n127 = call-poly <vilib>:"Mean.vi"("X"=w142) -> ("mean"=w151:dbl)  [unwired: 9 in, 1 out]
                    n128 = call-poly <vilib>:"Mean.vi"("X"=w163) -> ("mean"=w162:dbl)  [unwired: 9 in, 1 out]
                    n129 = Subtract(x=w141, y=w149) -> (x-y=w148:dbl[])
                    n130 = Subtract(x=w159, y=w165) -> (x-y=w164:dbl[])
                    n131 = local read "loopdiff2"() -> (w157:i64)
                    n132 = Subtract(x=w163, y=w162) -> (x-y=w161:dbl[])
                    n133 = Subtract(x=w152, y=w151) -> (x-y=w150:dbl[])
                    n134 = call-poly <vilib>:"Convolution.vi"("algorithm"=w147, "Y"=w148, "X"=w150) -> ("X * Y"=w146:dbl[])  [unwired: 7 in, 1 out]
                    n135 = call-poly <vilib>:"Convolution.vi"("algorithm"=w147, "Y"=w161, "X"=w164) -> ("X * Y"=w166:dbl[])  [unwired: 7 in, 1 out]
                    n136 = Array Max & Min(array=w146) -> (max index (indices)=w145:i32)  [unwired: 3 out]
                    n137 = Subtract(x=w145, y=w144) -> (x-y=w143:i32)
                    n138 = Array Max & Min(array=w166) -> (max index (indices)=w156:i32)  [unwired: 3 out]
                    n139 = Divide(x=w157, y=i64 5 ("x-y")) -> (x/y=w154:dbl)
                    n140 = Subtract(x=w156, y=w144) -> (x-y=w155:i32)
                    n141 = Compound Arithmetic op=ADD(w155, w143, w154) -> (w153:dbl)
                    n142 = local write "Latency Shift (Frames)"(w153) -> ()
                  }
                  frame #2 {
                    n143 = local write "Latency Check"(FALSE ("Latency Check")) -> ()
                  }
                }
              }
            }
          }
        }
      }
      n144 = node-c288(w20) -> ()  [unwired: 1 out]
    }
    frame #3 {
      w193 = u16 0 items=["DC", "Sine", "Square", "Triangle", "Ramp", "Pulse", "Noise", "Sinc", "Negative Ramp", "Exponential Rise", "Exponential Fall", "Cardiac"] ("Waveform Function (1: Sine)")
      # "Turn off ramp"
      n145 = local write "Z-ramp"(FALSE ("Z-ramp")) -> ()
      n146 = call "AG33_SetWaveform.vi"("Waveform Function (1: Sine)"=w193) -> ()  [unwired: 2 in, 1 out]
      n147 = property on="Z-ramp" class="Bool (strict)"("DisabledEnum"=T4."Enabled" ("Disabled")) -> ()  [unwired: 2 in, 2 out]
      n148 = call <vilib>:"DAQmx Clear Task.vi"("task in"=w191, "error in"=w190) -> ()  [unwired: 13 in, 1 out]
    }
  }
  n149 = stacked-sequence {
    seq-local: [_ _ _ _ w276 _ _] -> [_ _ _ _ _ w358 _]
    seq-local: [_ _ _ _ w277 _ _] -> [_ _ _ _ _ w361 _]
    seq-local: [_ _ _ _ w278 _ _] -> [_ _ _ _ _ w357 _]
    seq-local: [_ _ _ _ _ w360 _] -> [_ _ _ _ _ _ w504]
    seq-local: [_ _ _ _ _ w359 _] -> [_ _ _ _ _ _ w503]
    seq-local: [_ _ w263 _ _ _ _] -> [_ _ _ _ _ w344 _]
    seq-local: [_ _ _ w273 _ _ _] -> [_ _ _ _ _ w327 _]
    seq-local: [_ _ _ w272 _ _ _] -> [_ _ _ _ _ w343 _]
    seq-local: [_ _ w253 _ _ _ _] -> [_ _ _ _ _ w342 _]
    seq-local: [_ _ w241 _ _ _ _] -> [_ _ _ _ _ w338 _]
    seq-local: [_ _ _ _ w274 _ _] -> [_ _ _ _ _ w334 _]
    frame #0 {
      w197 = "O:\\"
      # "Make Dated and Time-stamped Directories"
      # "Setup File Paths"
      n150 = Format Date/Time String(time format string (%c)="%Y%m%d") -> (date/time string=w196:string)  [unwired: 2 in]
      n151 = Concatenate Strings(w197, w196, "\\Comments.txt" ("string")) -> (w194:string)
      n152 = String To Path(string=w194) -> (path=→"User Comments  File":path)
      n153 = Format Date/Time String(time format string (%c)="%Y%m%d_%H%M%S") -> (date/time string=w212:string)  [unwired: 2 in]
      n154 = local write "Comments"("") -> ()
      n155 = Concatenate Strings(w197, w196, "\\BrainScanner", w212) -> (w199:string)
      n156 = String To Path(string=w199) -> (path=w211:path)
      n157 = call <vilib>:"Check if File or Folder Exists.vi"("path"=w211) -> ("file or folder exists?"=w216:bool, "dup path"=w215:path)  [unwired: 8 in, 1 out]
      n158 = Concatenate Strings(w199, "\\CameraFrameData.txt" ("string")) -> (w203:string)
      n159 = Concatenate Strings(w199, "\\sCMOS_Frames_U16_1024x1024.dat" ("string")) -> (w208:string)
      n160 = Concatenate Strings(w199, "\\LabJackData.txt" ("string")) -> (w206:string)
      n161 = case shown="False" w216 {
        tunnel: [w218 w220] -> w210
        tunnel: w215 -> [w219 w220]
        frame False {
          n162 = Create Folder(path (use dialog)=w219) -> (created path=w218:path)  [unwired: 2 in, 2 out]
        }
        frame True {
        }
      }
      "Save Directory" <- w210
      n163 = String To Path(string=w203) -> (path=→"Camera Frame File":path)
      n164 = String To Path(string=w208) -> (path=→"sCMOS Camera Image File":path)
      n165 = String To Path(string=w206) -> (path=→"LabJack File":path)
    }
    frame #1 {
      # "Check to See if Motorized Focus Knob is Present"
      n166 = call "IsFocusControllerOn.vi"("VISA resource name"="Focus Knob COM Port") -> ("Succes"=w223:bool)  [unwired: 2 in, 2 out]
      n167 = case shown="True" w223 {
        selector: w223 -> [w224 _]
        tunnel: [w224 w225] -> w222
        tunnel: "Focus Knob COM Port" -> [_ w227]
        frame False {
        }
        frame True {
          # "Set Knob to Move slowly"
          n168 = call "SetupFocusKnobToMoveSlowly.vi"("VISA resource name"=w227, "Speed (higher is slower)"=255) -> ("Succes"=w225:bool)  [unwired: 2 in, 2 out]
        }
      }
      "Motorized Focus Knob Found" <- w222
    }
    frame #2 {
      w236 = "\r"
      w235 = "\t"
      w229 = "\t"
      # "Write File Headers"
      n169 = local read "Camera Frame File"() -> (w252:path)
      n170 = local read "LabJack File"() -> (w264:path)
      n171 = Open/Create/Replace File(file path (use dialog)=w252, operation (0:open)=T9."create", access (0:read/write)=enum16{"read/write", "read-only", "write-only"}."write-only") -> (refnum out=w262:refnum<file>, error out=w261:errorcluster)  [unwired: 3 in, 1 out]
      n172 = Open/Create/Replace File(file path (use dialog)=w264, operation (0:open)=T9."create", access (0:read/write)=enum16{"read/write", "read-only", "write-only"}."write-only") -> (refnum out=w269:refnum<file>, error out=w268:errorcluster)  [unwired: 3 in, 1 out]
      n173 = Concatenate Strings("Total Frames", w235, "Saved Frames", w235, "DC Offset", w235, "Image StDev", "\r") -> (w257:string)
      n174 = Concatenate Strings("FuncGen Voltage", w229, "Z Sensor", w229, "FxnGen Sync", w229, "Camera Trigger", w229, "Frame Count", w229, "Stage X" ("string"), w229, "Stage Y" ("string"), w229, "Photodiode" ("string"), "\r") -> (w267:string)
      n175 = Write to Text File(file (use dialog)=w262, text=w257, error in=w261) -> (refnum out=w253:refnum<file>)  [unwired: 1 in, 2 out]
      n176 = Write to Text File(file (use dialog)=w269, text=w267, error in=w268) -> (refnum out=w263:refnum<file>)  [unwired: 1 in, 2 out]
      n177 = local read "User Comments  File"() -> (w247:path)
      n178 = Open/Create/Replace File(file path (use dialog)=w247, operation (0:open)=T9."open or create", access (0:read/write)=enum16{"read/write", "read-only", "write-only"}."write-only") -> (refnum out=w244:refnum<file>)  [unwired: 3 in, 2 out]
      n179 = local read "Save Directory"() -> (w239:path)
      n180 = Set File Position(refnum=w244, from (0:start)=enum16{"start", "end", "current"}."end") -> (refnum out=w242:refnum<file>)  [unwired: 2 in, 1 out]
      n181 = Path To String(path=w239) -> (string=w238:string)
      n182 = Concatenate Strings(w236, w236, "---------------------  NEW FILE  ---------------------", w236, w238, w236, w236) -> (w237:string)
      n183 = Write to Text File(file (use dialog)=w242, text=w237) -> (refnum out=w241:refnum<file>)  [unwired: 2 in, 2 out]
      n184 = local write "Written"(w237) -> ()
    }
    frame #3 {
      # "Setup DAQ Streaming"
      n185 = call "DAQ Setup for Brain Imaging.vi"() -> ("error out"=w270:errorcluster, "task out"=w271:refnum<k21>)  [unwired: 10 in]
      n186 = call <vilib>:"DAQmx Start Task.vi"("task/channels in"=w271, "error in"=w270) -> ("task out"=w273:refnum<k21>, "error out"=w272:errorcluster)  [unwired: 12 in]
    }
    frame #4 {
      # "Initialize Camera"
      n187 = call <userlib>:"tm_initialize.vi"() -> ("error out"=w281:errorcluster, "Number Of Cameras"=w279:u32)  [unwired: 10 in]
      n188 = Not Equal To 0?(x=w279) -> (x != 0?=w280:bool)
      n189 = case shown="True" w280 {
        tunnel: w281 -> [_ w326]
        tunnel: [errorcluster {"status"=FALSE, "code"=0, "source"=""} ("error out") w294] -> w278
        tunnel: [u32 0 ("Handle out") w293] -> w276
        tunnel: [T10 {"height"=0, "width"=0, "datatype"=0} ("Buffer Info") w315] -> w277
        tunnel: [T3 {"Horizontal Offset"=0, "Vertical Offset"=0, "Horizontal Width"=0, "Vertical Width"=0} ("ROI") "ROI"] -> w274
        frame False {
          # "Abort if no camera found"
          n190 = Stop() -> ()  [unwired: 1 in]
        }
        frame True {
          w299 = "; " ("string")
          w313 = u32 6 items=["BINNING"=1, "BITS PER CHANNEL"=2, "ACTIVE VIEW INDEX"=3, "CCD MODE"=4, "SENSOR MODE"=5, "READOUT MODE"=6, "EXPOSURE TIME"=7, "CONTRAST GAIN"=8, "CONTRAST OFFSET"=9, "LIGHT MODE"=10, "SENSITIVITY"=11, "WHITE BALANCE"=12, "PHOTON IMAGING MODE"=13, "HIGH DYNAMIC RANGE MODE"=14, "TRIGGER SOURCE"=15, "TRIGGER ACTIVE"=16, "TRIGGER MODE"=17, "TRIGGER POLARITY"=18, "TRIGGER GLOBAL EXPOSURE"=19, "FIRST TRIGGER BEHAVIOR"=20, "TRIGGER TIMES"=21, "OUTPUT TRIGGER POLARITY"=22, "OUTPUT TRIGGER DELAY"=23, "OUTPUT TRIGGER PERIOD"=24, "TEMPERATURE"=25, "TEMPERATURE TARGET"=26, "SENSOR COOLER FAN"=27, "MECHANICAL SHUTTER"=28, "BACK FOCUS POSITION"=29, "FRAMEBUNDLE MODE"=30, "FRAMEBUNDLE NUMBER"=31, "LINEBUNDLE HEIGHT"=32, "TRIGGER CONNECTOR"=33, "IMAGE PIXEL TYPE"=34, "OUTPUT TRIGGER KIND"=35, "READOUT DIRECTION"=36, "CHANNEL SYNC"=37] ("Parameter")
          w316 = 1 items=["Snap", "Sequence"] ("Capture mode")
          w317 = u32 7 items=["BINNING"=1, "BITS PER CHANNEL"=2, "ACTIVE VIEW INDEX"=3, "CCD MODE"=4, "SENSOR MODE"=5, "READOUT MODE"=6, "EXPOSURE TIME"=7, "CONTRAST GAIN"=8, "CONTRAST OFFSET"=9, "LIGHT MODE"=10, "SENSITIVITY"=11, "WHITE BALANCE"=12, "PHOTON IMAGING MODE"=13, "HIGH DYNAMIC RANGE MODE"=14, "TRIGGER SOURCE"=15, "TRIGGER ACTIVE"=16, "TRIGGER MODE"=17, "TRIGGER POLARITY"=18, "TRIGGER GLOBAL EXPOSURE"=19, "FIRST TRIGGER BEHAVIOR"=20, "TRIGGER TIMES"=21, "OUTPUT TRIGGER POLARITY"=22, "OUTPUT TRIGGER DELAY"=23, "OUTPUT TRIGGER PERIOD"=24, "TEMPERATURE"=25, "TEMPERATURE TARGET"=26, "SENSOR COOLER FAN"=27, "MECHANICAL SHUTTER"=28, "BACK FOCUS POSITION"=29, "FRAMEBUNDLE MODE"=30, "FRAMEBUNDLE NUMBER"=31, "LINEBUNDLE HEIGHT"=32, "TRIGGER CONNECTOR"=33, "IMAGE PIXEL TYPE"=34, "OUTPUT TRIGGER KIND"=35, "READOUT DIRECTION"=36, "CHANNEL SYNC"=37] ("Parameter")
          w318 = u32 1 items=["BINNING"=1, "BITS PER CHANNEL"=2, "ACTIVE VIEW INDEX"=3, "CCD MODE"=4, "SENSOR MODE"=5, "READOUT MODE"=6, "EXPOSURE TIME"=7, "CONTRAST GAIN"=8, "CONTRAST OFFSET"=9, "LIGHT MODE"=10, "SENSITIVITY"=11, "WHITE BALANCE"=12, "PHOTON IMAGING MODE"=13, "HIGH DYNAMIC RANGE MODE"=14, "TRIGGER SOURCE"=15, "TRIGGER ACTIVE"=16, "TRIGGER MODE"=17, "TRIGGER POLARITY"=18, "TRIGGER GLOBAL EXPOSURE"=19, "FIRST TRIGGER BEHAVIOR"=20, "TRIGGER TIMES"=21, "OUTPUT TRIGGER POLARITY"=22, "OUTPUT TRIGGER DELAY"=23, "OUTPUT TRIGGER PERIOD"=24, "TEMPERATURE"=25, "TEMPERATURE TARGET"=26, "SENSOR COOLER FAN"=27, "MECHANICAL SHUTTER"=28, "BACK FOCUS POSITION"=29, "FRAMEBUNDLE MODE"=30, "FRAMEBUNDLE NUMBER"=31, "LINEBUNDLE HEIGHT"=32, "TRIGGER CONNECTOR"=33, "IMAGE PIXEL TYPE"=34, "OUTPUT TRIGGER KIND"=35, "READOUT DIRECTION"=36, "CHANNEL SYNC"=37] ("Parameter")
          w319 = u32 67109122 items=["BUS"=67109121, "CAMERA ID"=67109122, "VENDOR"=67109123, "MODEL"=67109124, "CAMERA VERSION"=67109125, "DRIVER VERSION"=67109126, "MODULE VERSIOIN"=67109127, "DCAMAPI VERSION"=67109128] ("Info ID")
          w321 = u32 67109125 items=["BUS"=67109121, "CAMERA"=67109122, "VENDOR"=67109123, "MODEL"=67109124, "CAMERA VERSION"=67109125, "DRIVER VERSION"=67109126, "MODULE VERSIOIN"=67109127, "DCAMAPI VERSION"=67109128] ("Info ID")
          w324 = u32 67109124 items=["BUS"=67109121, "CAMERA"=67109122, "VENDOR"=67109123, "MODEL"=67109124, "CAMERA VERSION"=67109125, "DRIVER VERSION"=67109126, "MODULE VERSIOIN"=67109127, "DCAMAPI VERSION"=67109128] ("Info ID")
          # "Start buffered acquisition"
          # "Setup Camera Trigger"
          # "Default 10 ms exp"
          # "Default 2x2 binning"
          n191 = call <userlib>:"tm_opencamera.vi"("error in (no error)"=w326, "Camera Index"=u32 0) -> ("error out"=w320:errorcluster, "Handle out"=w305:u32)  [unwired: 8 in]
          n192 = call <userlib>:"tm_getcamerainfo.vi"("error in (no error)"=w320, "Info ID"=w324, "Handle in"=w305) -> ("error out"=w323:errorcluster, "String"=w302:string)  [unwired: 6 in, 1 out]
          n193 = call <userlib>:"tm_getcamerainfo.vi"("error in (no error)"=w323, "Info ID"=w319, "Handle in"=w305) -> ("error out"=w322:errorcluster, "String"=w301:string)  [unwired: 6 in, 1 out]
          n194 = call <userlib>:"tm_getcamerainfo.vi"("error in (no error)"=w322, "Info ID"=w321, "Handle in"=w305) -> ("error out"=w304:errorcluster, "String"=w300:string)  [unwired: 6 in, 1 out]
          n195 = Concatenate Strings(w302, w299, w301, w299, w300) -> (→"Camera Info":string)
          n196 = local read "Binning"() -> (w296:u16)
          n197 = call <userlib>:"tm_setparameter.vi"("error in (no error)"=w304, "Value in"=2.0, "Parameter"=w313, "Handle in"=w305) -> ("error out"=w306:errorcluster, "Handle out"=w307:u32)  [unwired: 6 in]
          n198 = local read "Exposure (ms)"() -> (w295:dbl)
          n199 = call <userlib>:"tm_setparameter.vi"("error in (no error)"=w306, "Value in"=w296, "Parameter"=w318, "Handle in"=w307) -> ("error out"=w311:errorcluster, "Handle out"=w312:u32)  [unwired: 6 in]
          n200 = Divide(x=w295, y=1000.0) -> (x/y=w297:dbl)
          n201 = call <userlib>:"tm_setparameter.vi"("error in (no error)"=w311, "Value in"=w297, "Parameter"=w317, "Handle in"=w312) -> ("error out"=w292:errorcluster, "Handle out"=w291:u32)  [unwired: 6 in]
          n202 = call <userlib>:"tm_setarea.vi"("error in (no error)"=w292, "Sub Region"="ROI", "Handle in"=w291) -> ("error out"=w289:errorcluster, "Handle out"=w290:u32)  [unwired: 7 in]
          n203 = call <userlib>:"tm_setoutputtrigger.vi"("error in (no error)"=w289, "Parameters"=T11 {"Mode"=3, "Polarity"=2, "Period"=0.001, "Delay"=0.0}, "Handle in"=w290) -> ("error out"=w287:errorcluster, "Handle out"=w288:u32)  [unwired: 7 in]
          n204 = call <userlib>:"tm_preparecapture.vi"("error in (no error)"=w287, "Capture mode"=w316, "Handle in"=w288) -> ("error out"=w309:errorcluster, "Buffer Info"=w315:T10, "Handle out"=w310:u32)  [unwired: 5 in, 1 out]
          n205 = call <userlib>:"tm_startcapture_b.vi"("error in (no error)"=w309, "Handle in"=w310) -> ("error out"=w294:errorcluster, "Handle out"=w293:u32)  [unwired: 8 in]
        }
      }
      n206 = local write "Quit Pushed?"(FALSE ("stop")) -> ()
    }
    frame #5 {
      w336 = 0
      # "Made this 80 ms with priority of 2 --Andy 6/4/2015"
      # "Run Main Camera and DAQ Loops"
      n207 = node-c288() -> (w349:T5)  [unwired: 4 in]
      n208 = Unbundle By Name(w334) -> ("Horizontal Width"=w333:i32, "Vertical Width"=w332:i32)
      n209 = local read "sCMOS Camera Image File"() -> (w356:path)
      n210 = timed-loop {
        timing: w349 -> [_]
        timing-out: [_] -> w348
        tunnel: w327 -> [w417]
        tunnel: w343 -> [w416]
        tunnel: [w423] -> w347
        tunnel: w344 -> [w422]
        tunnel: [w415] -> w331
        tunnel: [w414] -> w330
        stop <- w418 stop-if-true
        # "DAQ Stream to Disk"
        n211 = node-c288() -> ()  [unwired: 1 in, 1 out]
        n212 = local read "output cluster"() -> (w402:T2)
        n213 = local read "Saved Images Hidden"() -> (w412:i32)
        n214 = call-poly <vilib>:"DAQmx Read.vi"("task/channels in"=w417, "error in"=w416) -> ("task out"=w415:refnum<k21>, "data"=w407:dbl[], "error out"=w414:errorcluster)  [unwired: 11 in]
        n215 = local read "Stage X"() -> (w410:i32)
        n216 = local read "Stage Y"() -> (w409:i32)
        n217 = Tick Count (ms)() -> (millisecond timer value=w403:u32)
        n218 = local read "TotalFramesHidden"() -> (w411:i32)
        n219 = local read "Quit Pushed?"() -> (w418:bool)
        n220 = Unbundle(w402) -> ("Actual Start [i]"=w405:i64, "standard deviation"=w400:dbl)
        n221 = Index Array(array=w407, index=4) -> (element=w399:dbl)
        "photodiode" <- w399
        n222 = Index Array(array=w407, index=1 ("index (row)")) -> (element=w408:dbl)
        "FuncGen Voltage" <- w408
        n223 = Index Array(array=w407, index=2 ("index (row)")) -> (element=w419:dbl)
        "Camera Trigger" <- w419
        n224 = Index Array(array=w407, index=0 ("index (row)")) -> (element=w421:dbl)
        "Z Sensor" <- w421
        n225 = Index Array(array=w407, index=3 ("index (row)")) -> (element=w420:dbl)
        "FxnGen Sync" <- w420
        n226 = Subtract(x=w403, y=w405) -> (x-y=→"loopdiff2":i64)
        n227 = Bundle("standard deviation"=w400, "Waveform"=w399) -> (→"output cluster 2":T14)  [unwired: 1 in]
        n228 = call "MakeLabJackString.vi"("FuncGen Voltage"=w408, "X position"=w410, "Z Sensor"=w421, "FxnGen Sync"=w420, "Y position"=w409, "Camera Trigger"=w419, "Total Frame Count"=w411, "Save Image Counts"=w412) -> ("Output String"=w424:string)  [unwired: 11 in]
        n229 = node-c288() -> ()  [unwired: 1 in, 1 out]
        n230 = Write to Text File(file (use dialog)=w422, text=w424) -> (refnum out=w423:refnum<file>)  [unwired: 2 in, 2 out]
      }
      n231 = Open/Create/Replace File(file path (use dialog)=w356, operation (0:open)=T9."create", access (0:read/write)=enum16{"read/write", "read-only", "write-only"}."write-only") -> (refnum out=w355:refnum<file>)  [unwired: 3 in, 2 out]
      n232 = Tick Count (ms)() -> (millisecond timer value=w362:u32)
      n233 = Multiply(x=w333, y=w332) -> (x*y=w335:i32)
      n234 = node-c288() -> (w353:T5)  [unwired: 4 in]
      n235 = timed-loop "Timed Loop" {
        tunnel: w357 -> [w468]
        tunnel: [w466] -> w360
        tunnel: [w465] -> w359
        tunnel: w358 -> [w469]
        tunnel: w362 -> [w470]
        shift-right: [w446] -> _
        shift-left: w336 -> [w440]
        tunnel: w355 -> [w458]
        tunnel: [w457] -> w354
        timing: w353 -> [_]
        timing-out: [_] -> w352
        tunnel: w361 -> [w464]
        tunnel: w342 -> [w453]
        tunnel: [w452] -> w341
        shift-right: [w445] -> _
        shift-left: w336 -> [w448]
        tunnel: w335 -> [w443]
        i -> [w463]
        stop <- w449 stop-if-true
        # "Camera and File Control Loop"
        n236 = node-c288() -> ()  [unwired: 1 in, 1 out]
        n237 = Increment(x=w448) -> (x+1=w445:i32)
        n238 = call <userlib>:"tm_waitnextframe.vi"("error in (no error)"=w468, "Handle in"=w469) -> ("error out"=w462:errorcluster, "Frame Count"=w435:i32, "Frame Index"=w455:i32, "Handle out"=w461:u32)  [unwired: 6 in]
        "TotalFramesHidden" <- w435
        n239 = Tick Count (ms)() -> (millisecond timer value=w467:u32)
        n240 = call <userlib>:"tm_getframe_a.vi"("error in (no error)"=w462, "Frame Index"=w455, "Buffer Info"=w464, "Handle in"=w461) -> ("error out"=w465:errorcluster, "Data 16"=w438:u16[][], "Handle out"=w466:u32)  [unwired: 3 in, 2 out]
        n241 = Subtract(x=w467, y=w470) -> (x-y=w456:u32)
        n242 = Reshape Array(w438, w443) -> (w444:u16[])
        n243 = Quotient & Remainder(x=w463, y=20) -> (x-y*floor(x/y)=w459:i32)  [unwired: 1 out]
        n244 = Equal To 0?(x=w459) -> (x = 0?=w454:bool)
        n245 = case shown="1" "AutoFocus" {
          tunnel: w438 -> [w471 w475 w479]
          tunnel: [w471 w474 w476] -> w437
          frame 0, Default {
          }
          frame 1 {
            w472 = 600 ("length")
            w473 = 0 ("index")
            n246 = Array Subset(array=w475, index (row)=w473, length (row)=w472, index (col)=w473, length (col)=w472) -> (w474:u16[][])
          }
          frame 2 {
            w477 = 600 ("index")
            n247 = Array Subset(array=w479, index (row)=0 ("index"), length (row)=w477, index (col)=w477, length (col)=w477) -> (w476:u16[][])
          }
        }
        n248 = case shown="True" w454 {
          tunnel: w456 -> [_ w496]
          tunnel: w435 -> [_ w494]
          tunnel: w440 -> [_ w492]
          tunnel: w438 -> [_ w493]
          tunnel: w445 -> [_ w491]
          frame False {
          }
          frame True {
            n249 = Subtract(x=w494, y=w491) -> (x-y=→"Dropped Frames":i32)
            n250 = Divide(x=w496, y=u32 1000) -> (x/y=w498:dbl)
            n251 = call "Seconds to HMS.vi"("Time Elapsed in Seconds"=w498) -> ("Time Elapsed (H : M : S)"=→"Elapsed Time":string)
            "Total Frames" <- w494
            "Current Image" <- w493
            "Saved Frames" <- w492
            "Read Frames" <- w491
          }
        }
        n252 = Reshape Array(w437, 360000 ("index")) -> (w442:u16[])
        n253 = local read "Z-ramp DC Offset"() -> (w450:dbl)
        n254 = Decimate 1D Array(w442) -> (w436:u16[])  [unwired: 33 out]
        n255 = call <vilib>:"Std Deviation and Variance.vi"("X"=w436) -> ("standard deviation"=w434:dbl)  [unwired: 1 in, 2 out]
        "Image StDev" <- w434
        n256 = local read "Save Image"() -> (w447:bool)
        n257 = Tick Count (ms)() -> (millisecond timer value=w433:u32)
        n258 = local read "Quit Pushed?"() -> (w449:bool)
        n259 = call "MakeCameraDataString.vi"("Image StDev"=w434, "DC Offset"=w450, "Saved Frame Number"=w440, "Frame Number"=w435) -> ("Output String"=w451:string)
        n260 = Bundle("millisecond timer value"=w433, "standard deviation"=w434) -> (→"output cluster":T15)  [unwired: 1 in]
        n261 = Write to Text File(file (use dialog)=w453, text=w451) -> (refnum out=w452:refnum<file>)  [unwired: 2 in, 2 out]
        n262 = case shown="True" w447 {
          tunnel: w458 -> [w481 w488]
          tunnel: [w481 w487] -> w457
          tunnel: w444 -> [_ w486]
          tunnel: w440 -> [w480 w483]
          tunnel: [w480 w482] -> w446
          frame False {
          }
          frame True {
            n263 = Increment(x=w483) -> (x+1=w482:i32)
            n264 = Write to Binary File(file (use dialog)=w488, data=w486, 5:FALSE ("prepend array or string size? (T)"), 9:T13."little-endian" ("byte order (0:big-endian, network order)")) -> (refnum out=w487:refnum<file>)  [unwired: 2 in, 2 out]
          }
        }
        n265 = node-c288() -> ()  [unwired: 1 in, 1 out]
        "Saved Images Hidden" <- w440
      }
      n266 = node-c288(w348) -> ()
      n267 = call <vilib>:"DAQmx Clear Task.vi"("task in"=w331, "error in"=w330) -> ()  [unwired: 13 in, 1 out]
      n268 = Close File(refnum=w347) -> ()  [unwired: 1 in, 2 out]
      n269 = node-c288() -> (w329:T5)  [unwired: 4 in]
      n270 = node-c288() -> (w346:T5)  [unwired: 2 in]
      n271 = timed-loop {
        timing: w329 -> [_]
        timing-out: [_] -> w328
        stop <- w365 stop-if-true
        n272 = node-c288() -> ()  [unwired: 1 in, 1 out]
        n273 = call "WHERE_XY_Parsed fast_20141209_FBS.vi"() -> ("X"=→"Stage X":i32, "Y"=→"Stage Y":i32)  [unwired: 1 in, 2 out]
        n274 = local read "Quit Pushed?"() -> (w365:bool)
        n275 = node-c288() -> ()  [unwired: 1 in, 1 out]
      }
      n276 = timed-loop {
        timing: w346 -> [_]
        timing-out: [_] -> w345
        stop <- "Quit" stop-if-true
        # "Update Image Display"
        n277 = node-c288() -> ()  [unwired: 1 in, 1 out]
        n278 = local read "Current Image"() -> (w392:u16[][])
        n279 = call "Bin 2D Array.vi"("Input Array"=w392, "Binning Value"=u8 3) -> ("Binned Array"=→"sCMOS Image":u16[][])
        n280 = node-c288() -> ()  [unwired: 1 in, 1 out]
        "Quit Pushed?" <- "Quit"
      }
      n281 = node-c288(w328) -> ()  [unwired: 1 out]
      n282 = node-c288(w345) -> ()
      n283 = node-c288() -> (w340:T5)  [unwired: 2 in]
      n284 = timed-loop {
        timing: w340 -> [_]
        timing-out: [_] -> w339
        tunnel: w338 -> [w371]
        tunnel: [w371] -> w337
        stop <- w372 stop-if-true
        # "Comment File Update"
        n285 = node-c288() -> ()  [unwired: 1 in]
        n286 = event shown="[1] \"Comments\": Key Down" {
          selector: _ -> [_ _]
          dyn-events: _ -> [_ _]
          timeout: 0 -> [_ _]
          tunnel: w371 -> [_ w373]
          event Timeout {
            n287 = event-data() -> ()  [unwired: 1 in, 3 out]
          }
          event "Comments": Key Down {
            # "Write to file if return pressed"
            n288 = event-data() -> ("VKey"=w376:T12)  [unwired: 1 in, 1 out]
            n289 = Equal?(x=w376, y=eventvkey."Return") -> (x = y?=w374:bool)
            n290 = case shown="True" w374 {
              tunnel: w373 -> [_ w378]
              frame False {
              }
              frame True {
                n291 = flat-sequence {
                  tunnel: w378 -> [w381]
                  tunnel: [w380] -> w377
                  tunnel: w377 -> [w383]
                  frame #0 {
                    n292 = local read "Comments"() -> (w379:string)
                    n293 = call "MakeCommentString.vi"("Input string"=w379) -> ("Output String"=w380:string)
                    n294 = Write to Text File(file (use dialog)=w381, text=w380) -> ()  [unwired: 2 in, 3 out]
                  }
                  frame #1 {
                    n295 = local read "Written"() -> (w384:string)
                    n296 = Concatenate Strings(w384, w383) -> (→"Written":string)
                  }
                  frame #2 {
                    n297 = local write "Comments"("") -> ()
                    n298 = property on="Written" class="Str"("Text.Scroll Position"=-1) -> ()  [unwired: 2 in, 2 out]
                  }
                }
              }
            }
          }
        }
        n299 = local read "Quit Pushed?"() -> (w372:bool)
        n300 = node-c288() -> ()  [unwired: 1 out]
      }
      n301 = node-c288 ("Output Node")(w352) -> ()  [unwired: 1 out]
      n302 = Close File(refnum=w341) -> ()  [unwired: 1 in, 2 out]
      n303 = node-c288(w339) -> ()
      n304 = Close File(refnum=w354) -> ()  [unwired: 1 in, 2 out]
      n305 = Close File(refnum=w337) -> ()  [unwired: 1 in, 2 out]
    }
    frame #6 {
      # "Close Camera"
      n306 = local write "Motorized Focus Knob Found"(FALSE ("Motorized Focus Knob Found")) -> ()
      n307 = call <userlib>:"tm_stopcapture.vi"("error in (no error)"=w503, "Handle in"=w504) -> ("error out"=w506:errorcluster)  [unwired: 8 in, 1 out]
      n308 = call <userlib>:"tm_unpreparecapture.vi"("error in (no error)"=w506) -> ("error out"=w505:errorcluster)  [unwired: 9 in, 1 out]
      n309 = call <userlib>:"tm_closecamera.vi"("error in (no error)"=w505) -> ("error out"=w507:errorcluster)  [unwired: 10 in]
      n310 = call <userlib>:"tm_deinitialize.vi"("error in (no error)"=w507) -> ()  [unwired: 10 in, 1 out]
    }
  }
